vi "General_Monitoring_rt_v2.vi"() -> ()   [LabVIEW 2014]
uses:
  <vilib>/Utility/RT CPU Load.ctl
  <vilib>/Platform/TimedLoop/XDataNode/timing_clust.ctl
  <vilib>/Platform/TimedLoop/XDataNode/nitl_modes.ctl
  <vilib>/Platform/TimedLoop/XDataNode/wakeup.ctl
  <vilib>/platform/TimedLoop/XDataNode/XDataNode.xnode
  <vilib>/Platform/TimedLoop/XDataNode/XDNodeRunTimeDep.lvlib
  <vilib>/NI_Real-Time Target Support.lvlib
panel:
  in  "Flight Number":string
  out "PRTAFT_UDP_In 2":string
  out "Disconnect Watchdog":bool
  out "Disk Space Used %":dbl
  out "Synced?":bool
  out "Clock_ID":string
  out "AI0":dbl
  out "CPU Load Total":dbl
  out "CPU loads":T1[](array[typedef]) {"ISR (%)" format="%#.2f"; "Idle (%)" format="%#.2f"; "Background (%)" format="%#.2f"; "Normal (%)" format="%#.2f"; "Above Normal (%)" format="%#.2f"; "High (%)" format="%#.2g"; "Timed Structures (%)" format="%#.2g"; "Time Critical (%)" format="%#.2g"; "Total (%)" format="%#.2g"}
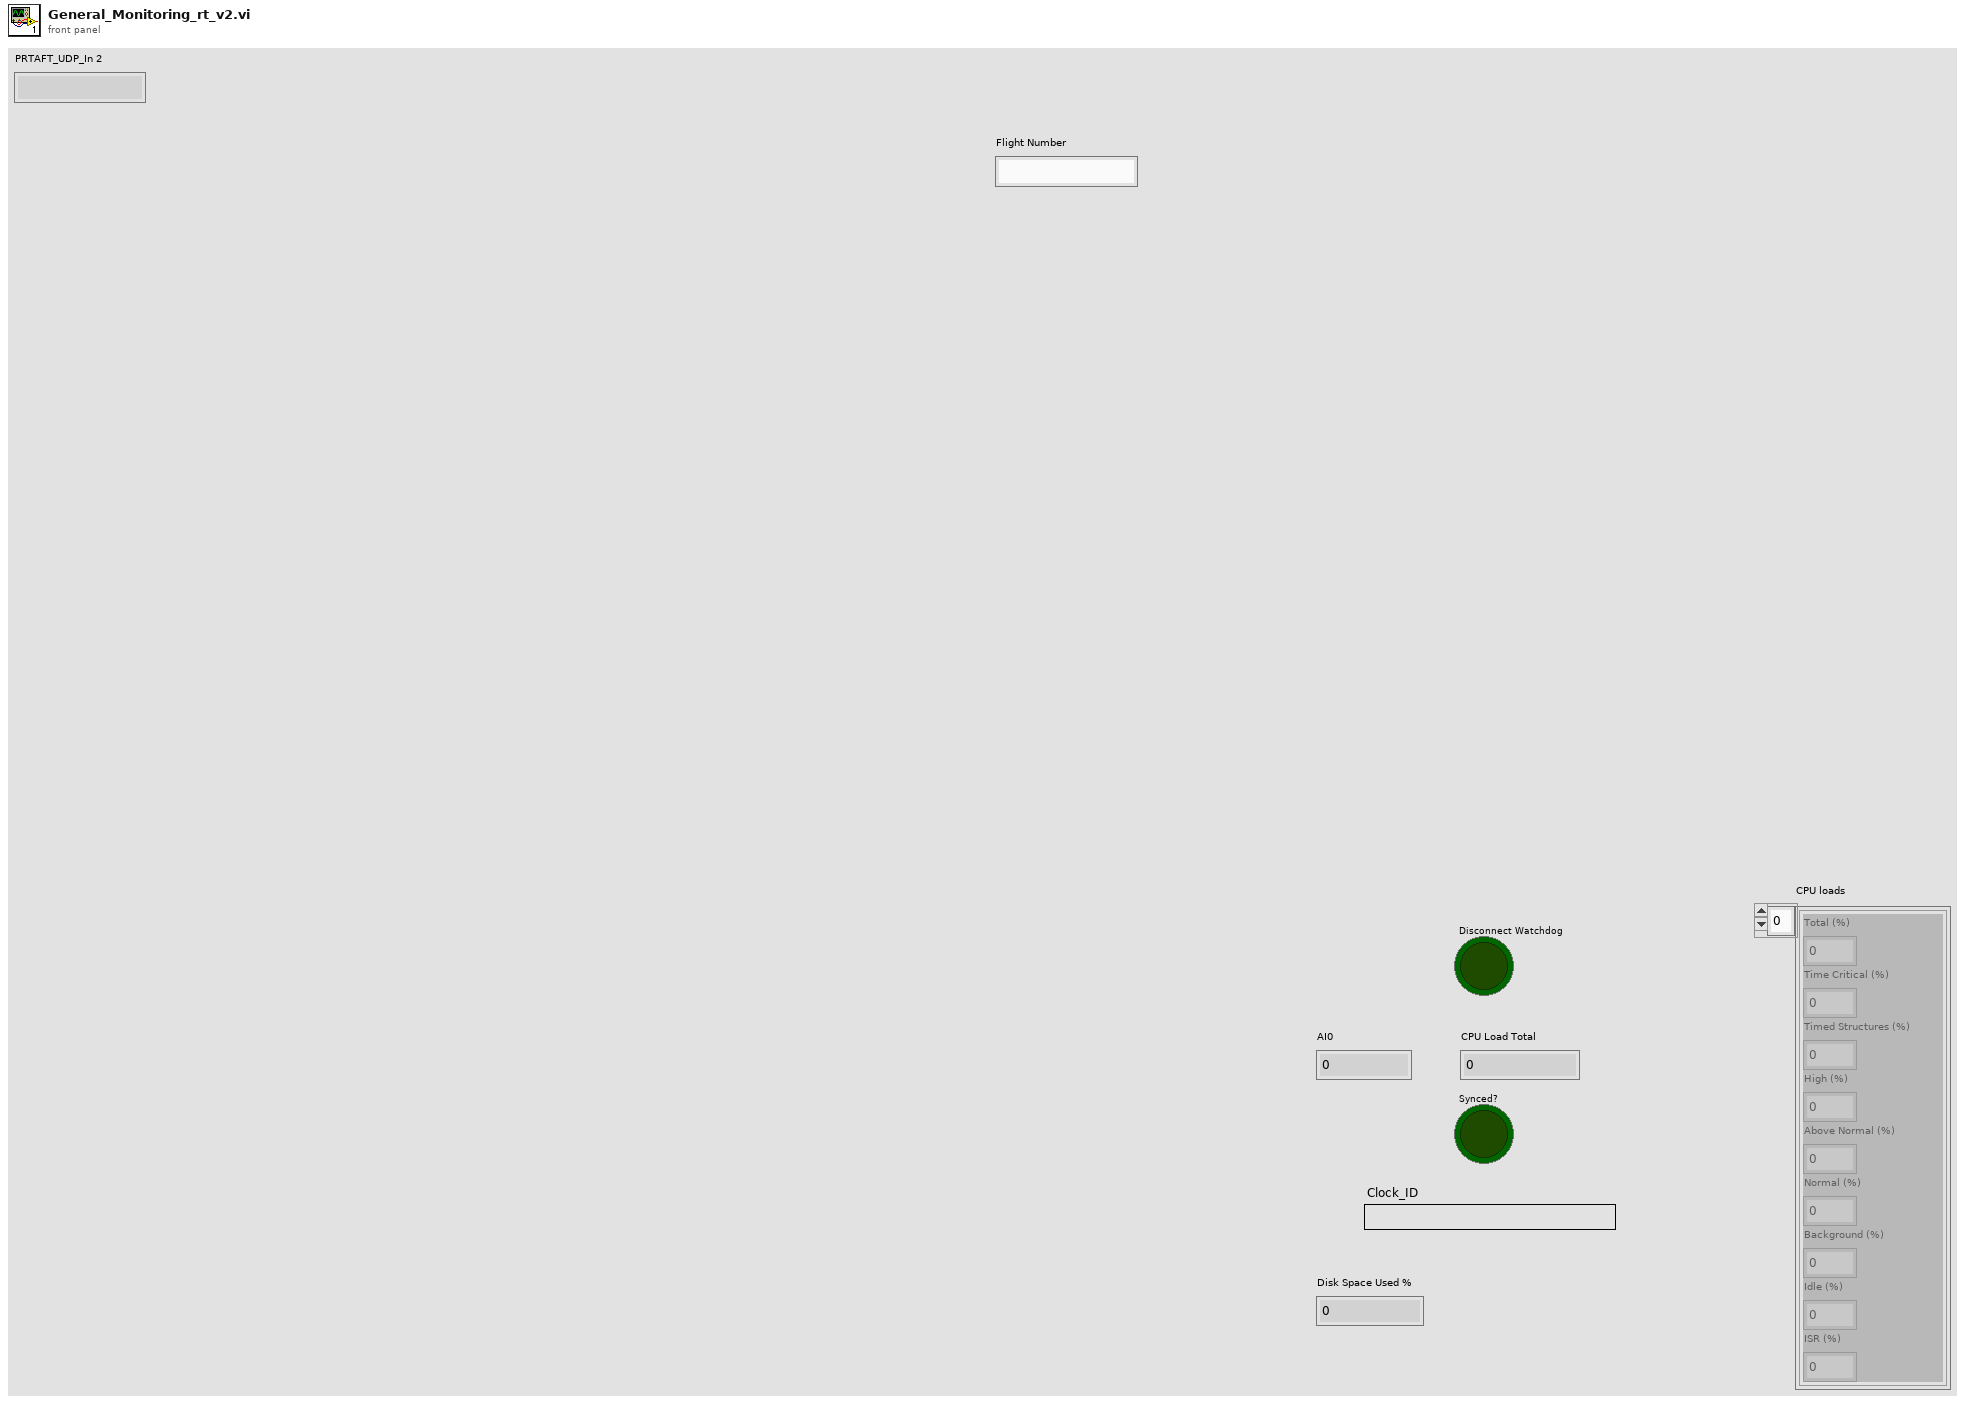
[diagram p1: front panel]
types:
  T1 = typedef "NI_Real-Time Target Support.lvlib/RT CPU Load.ctl" = cluster{"Total (%)":dbl, "Time Critical (%)":dbl, "Timed Structures (%)":dbl, "High (%)":dbl, "Above Normal (%)":dbl, "Normal (%)":dbl, "Background (%)":dbl, "Idle (%)":dbl, "ISR (%)":dbl}
  T2 = typedef "XDNodeRunTimeDep.lvlib/timing_clust.ctl" = cluster{"Expected End [f-1]":u64, "Actual End [f-1]":u64, "Finished Late? [f-1]":bool, "Expected End [i-1]":u64, "Actual End [i-1]":u64, "Finished Late? [i-1]":bool, "Expected Start [i]":u64, "Actual Start [i]":u64, "Expected Start [f]":u64, "Actual Start [f]":u64, "Source Name":string, "Structure Name":string, "Period":i64, "Deadline":i64, "Offset":i64, "Start":i64, "Priority":i32, "Timeout":i32, "Mode":T3, "Wakeup Reason":T4, "Error":errorcluster, "Source Type":string, "Secondary Source Type":string, "Global End Time":u64, "Global Start Time":u64, "Frame Duration":u64, "Iteration Duration":u64, "Assigned CPU":i32, "I/O Scan Engine Mode":u32}
  T3 = typedef "XDNodeRunTimeDep.lvlib/nitl_modes.ctl" = enum32{"No Change", "Process missed periods, maintain original phase", "Discard missed periods, maintain original phase", "Process missed periods, ignore original phase", "Discard missed periods, ignore original phase"}
  T4 = typedef "XDNodeRunTimeDep.lvlib/wakeup.ctl" = enum32{"Normal", "Aborted", "Asynchronous wakeup", "Timing source error", "Timed loop error", "Timeout"}
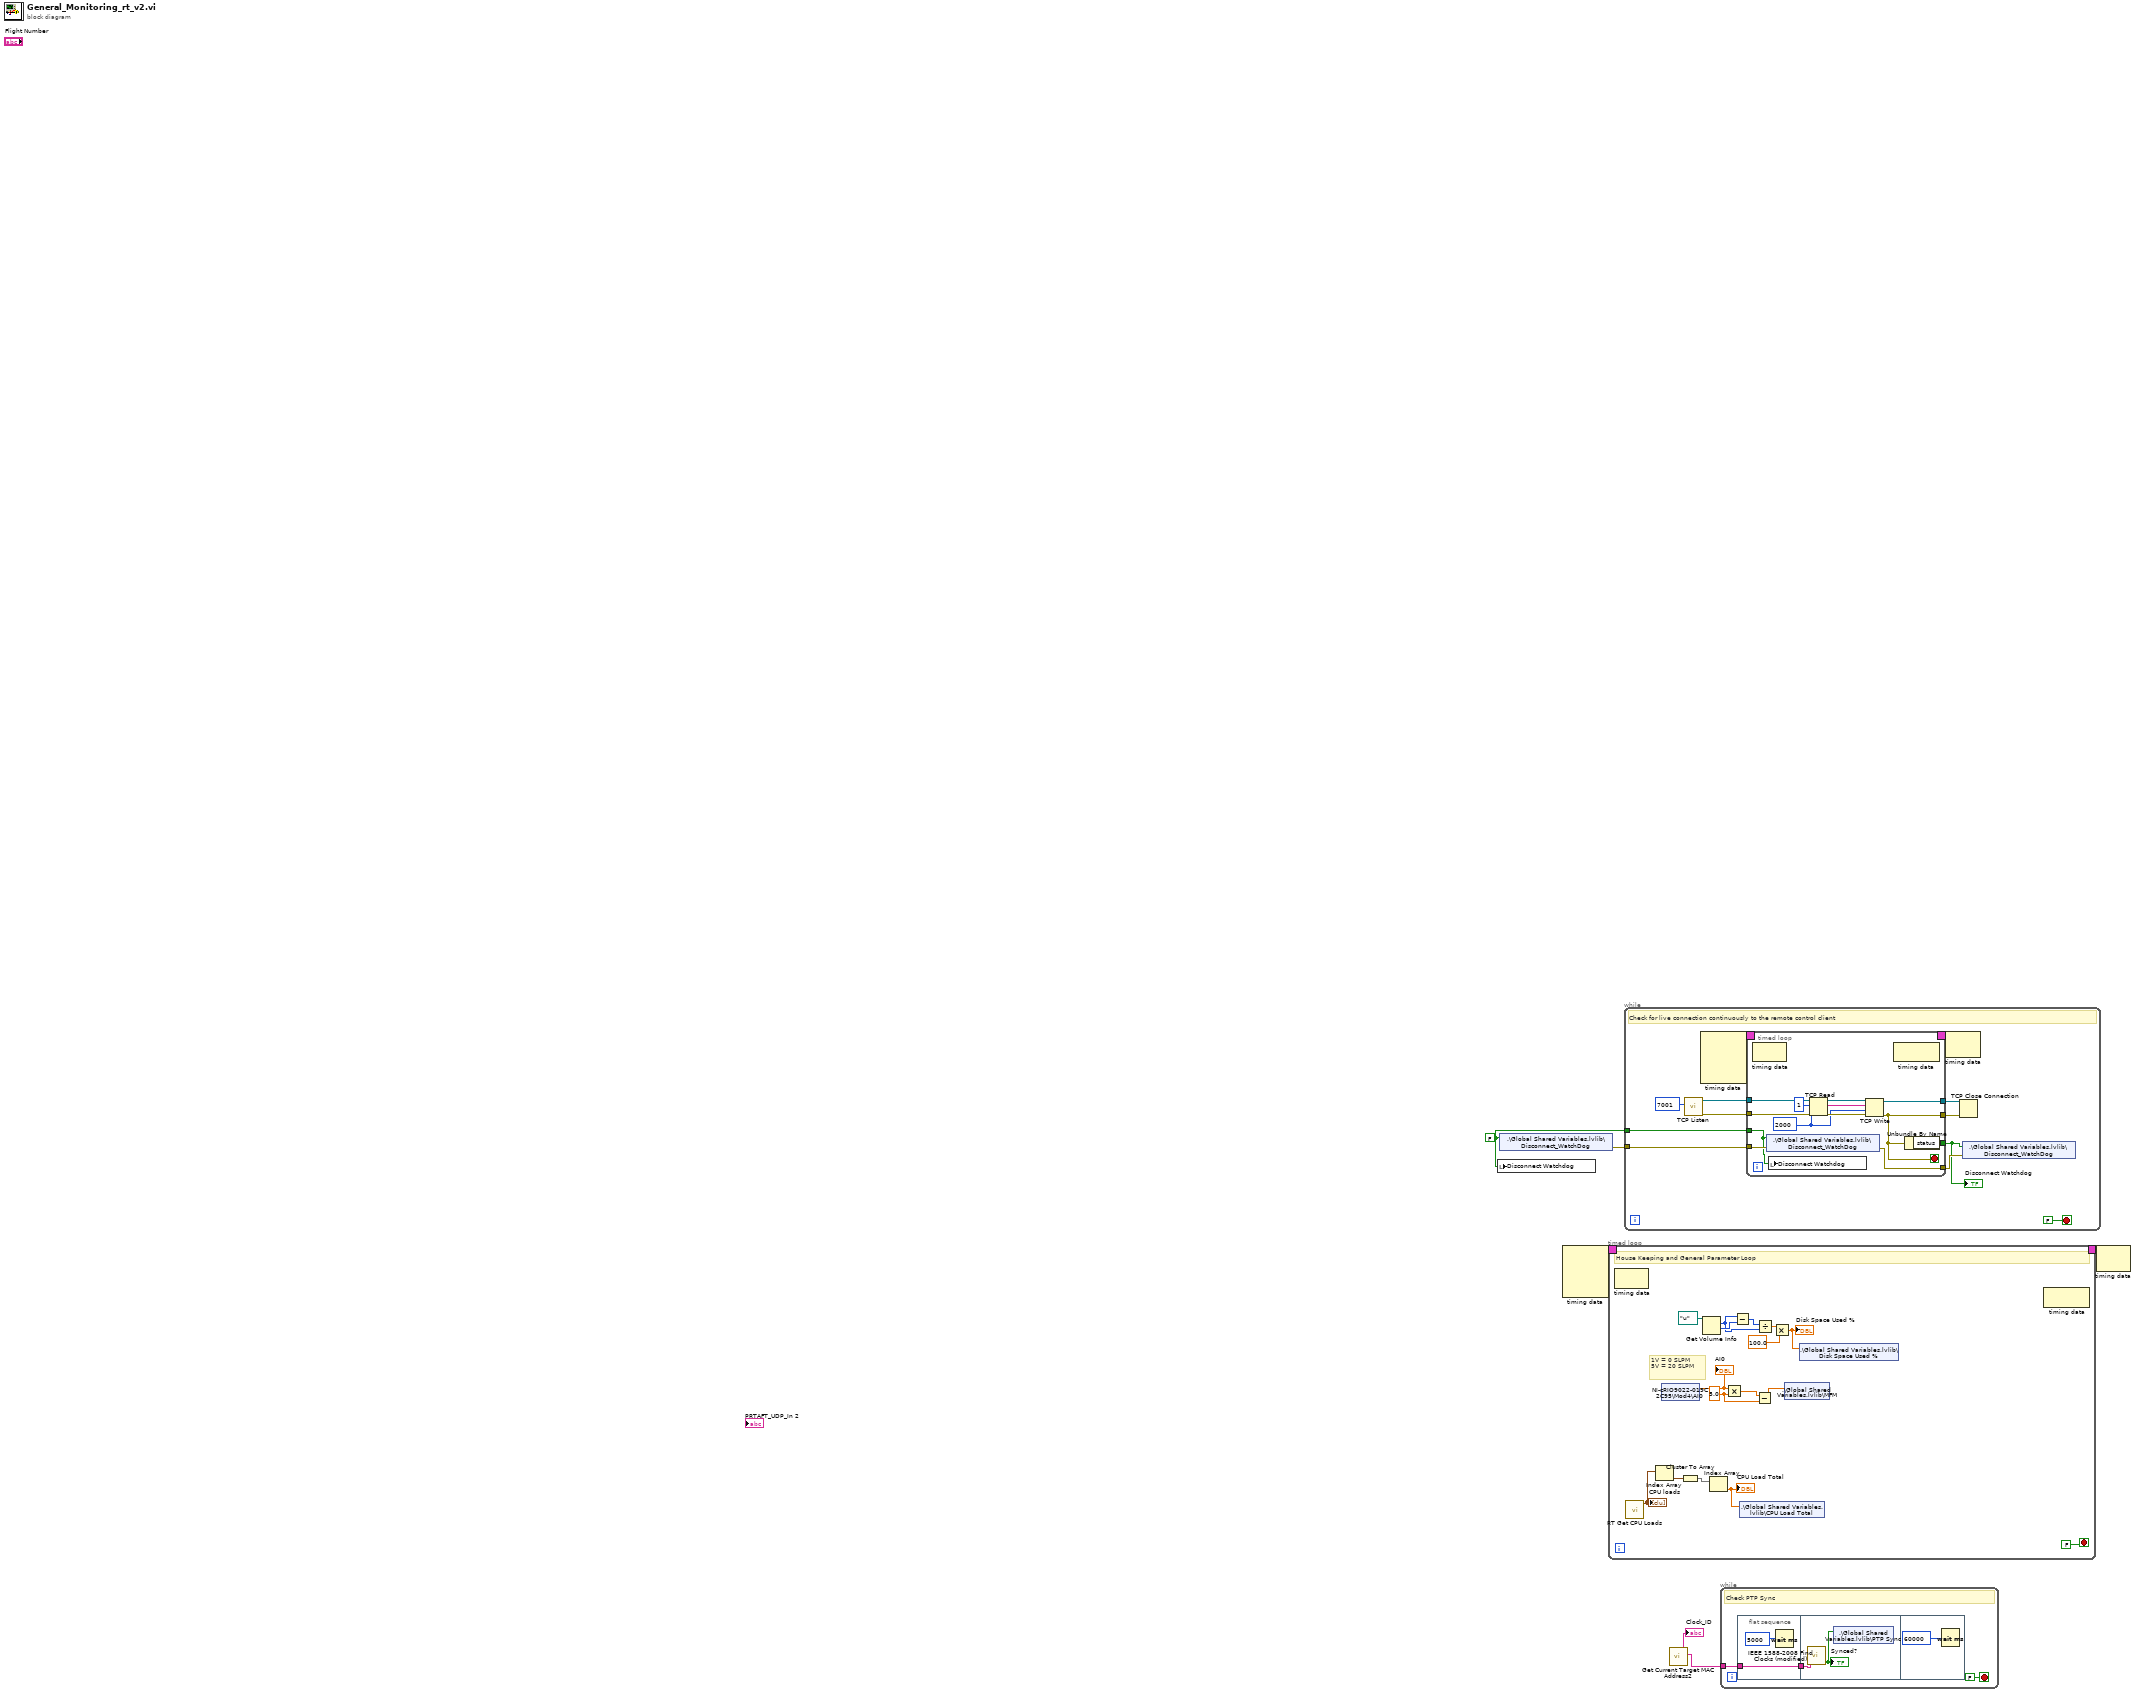
[diagram p0: block diagram]
diagram:
  w1 = FALSE ("Connect_WatchDog")
  n1 = local write "Disconnect Watchdog"(w1) -> ()
  n2 = shared-variable ".\\Global Shared Variables.lvlib\\Disconnect_WatchDog"(w1) -> (error out=w2:errorcluster)  [unwired: 1 in]
  n3 = node-c288() -> (w5:T2)  [unwired: 4 in]
  n4 = timed-loop {
    timing: w5 -> [_]
    timing-out: [_] -> w4
    stop <- FALSE stop-if-true
    w13 = 5.0 ("y")
    # "1V = 0 SLPM\n5V = 20 SLPM"
    # "House Keeping and General Parameter Loop"
    n5 = node-c288() -> ()  [unwired: 1 in, 1 out]
    n6 = call <vilib>:"RT Get CPU Loads.vi"() -> ("CPU loads"=w21:T1[])  [unwired: 10 in, 1 out]
    "CPU loads" <- w21
    n7 = Index Array(array=w21) -> (element=w20:T1)  [unwired: 1 in]
    n8 = shared-variable "NI-cRIO9022-019C2C95\\Mod4\\AI0"() -> (w16:dbl)  [unwired: 1 in, 1 out]
    "AI0" <- w16
    n9 = Cluster To Array(cluster=w20) -> (array=w18:dbl[])
    n10 = Get Volume Info(11:path "u:/" ("path")) -> (1:w11:i64, 2:w9:i64)  [unwired: 1 in, 4 out]
    n11 = Index Array(array=w18) -> (element=w17:dbl)  [unwired: 1 in]
    "CPU Load Total" <- w17
    n12 = Multiply(x=w16, y=w13) -> (x*y=w14:dbl)
    n13 = Subtract(x=w9, y=w11) -> (x-y=w10:i64)
    n14 = shared-variable ".\\Global Shared Variables.lvlib\\CPU Load Total"(w17) -> ()  [unwired: 1 in, 1 out]
    n15 = Subtract(x=w14, y=w13) -> (x-y=w15:dbl)
    n16 = Divide(x=w10, y=w9) -> (x/y=w8:dbl)
    n17 = Multiply(x=w8, y=100.0) -> (x*y=w6:dbl)
    "Disk Space Used %" <- w6
    n18 = shared-variable ".\\Global Shared Variables.lvlib\\MFM"(w15) -> ()  [unwired: 1 in, 1 out]
    n19 = shared-variable ".\\Global Shared Variables.lvlib\\Disk Space Used %"(w6) -> ()  [unwired: 1 in, 1 out]
    n20 = node-c288() -> ()  [unwired: 1 in, 1 out]
  }
  n21 = while {
    tunnel: w1 -> [w29]
    tunnel: w2 -> [w28]
    stop <- FALSE stop-if-true
    # "Check for live connection continuously to the remote control client"
    n22 = call <vilib>:"TCP Listen.vi"("port"=u16 7001) -> ("error out"=w35:errorcluster, "connection ID"=w34:refnum<k5>)  [unwired: 6 in, 3 out]
    n23 = node-c288() -> (w25:T2)  [unwired: 4 in]
    n24 = timed-loop {
      tunnel: w35 -> [w47]
      tunnel: w34 -> [w48]
      tunnel: [w42] -> w26
      tunnel: [w41] -> w31
      tunnel: [w40] -> w30
      tunnel: w29 -> [w37]
      tunnel: w28 -> [w39]
      tunnel: [w38] -> w27
      timing: w25 -> [_]
      timing-out: [_] -> w24
      stop <- w41 stop-if-true
      w36 = 2000 ("timeout ms (25000)")
      n25 = node-c288() -> ()  [unwired: 1 in, 1 out]
      n26 = shared-variable ".\\Global Shared Variables.lvlib\\Disconnect_WatchDog"(w37, error in=w39) -> (error out=w38:errorcluster)
      n27 = local write "Disconnect Watchdog"(w37) -> ()
      n28 = TCP Read(connection ID=w48, bytes to read=1, error in (no error)=w47, 9:w36) -> (connection ID out=w45:refnum<k5>, data out=w43:string, error out=w44:errorcluster)  [unwired: 1 in]
      n29 = TCP Write(connection ID=w45, data in=w43, error in (no error)=w44, 9:w36) -> (connection ID out=w40:refnum<k5>, error out=w41:errorcluster)  [unwired: 1 out]
      n30 = node-c288() -> ()  [unwired: 1 in, 1 out]
      n31 = Unbundle By Name(w41) -> ("status"=w42:bool)
    }
    "Disconnect Watchdog" <- w26
    n32 = node-c288(w24) -> ()  [unwired: 1 out]
    n33 = TCP Close Connection(connection ID=w30, error in (no error)=w31) -> ()  [unwired: 1 in, 2 out]
    n34 = shared-variable ".\\Global Shared Variables.lvlib\\Disconnect_WatchDog"(w26, error in=w27) -> ()  [unwired: 1 out]
  }
  n35 = call "Get Current Target MAC Address2.vi"() -> ("Clock_ID"=w3:string)  [unwired: 9 in, 2 out]
  "Clock_ID" <- w3
  n36 = while {
    tunnel: w3 -> [w55]
    stop <- FALSE stop-if-true
    # "Check PTP Sync"
    n37 = flat-sequence {
      tunnel: w55 -> [w57]
      tunnel: [w57] -> w54
      tunnel: w54 -> [w59]
      frame #0 {
        n38 = Wait (ms)(milliseconds to wait=u32 5000) -> ()  [unwired: 1 out]
      }
      frame #1 {
        n39 = call "IEEE 1588-2008 Find Clocks (modified).vi"("Clock Id to Verify"=w59) -> ("Synced?"=w58:bool)  [unwired: 10 in]
        "Synced?" <- w58
        n40 = shared-variable ".\\Global Shared Variables.lvlib\\PTP Sync"(w58) -> ()  [unwired: 1 in, 1 out]
      }
      frame #2 {
        n41 = Wait (ms)(milliseconds to wait=u32 60000) -> ()  [unwired: 1 out]
      }
    }
  }
  n42 = node-c288(w4) -> ()  [unwired: 1 out]
